vi "Read Input Registers.vi"(8 "error in (no error)":errorcluster, 9 "number of input registers":u16, 10 "address":u16, 11 "MODBUS in":refnum<class "PL Modbus Client.lvclass">) -> (0 "error out":errorcluster, 2 "values":u16[](array[numeric]), 3 "MODBUS out":refnum<class "PL Modbus Client.lvclass">)   [LabVIEW 2015, in "PL Modbus Client.lvclass"]
doc: "Reads a specified <B>number of input registers</B> starting at specified <B>address</B> (Modbus function code: <B>4</B>)."
uses:
  PL Modbus Client.lvclass
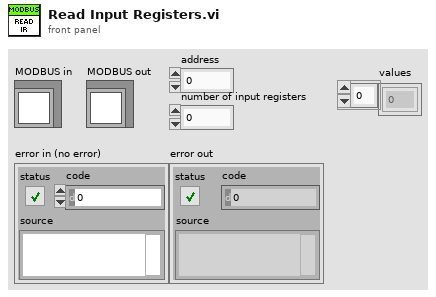
[diagram p1: front panel]
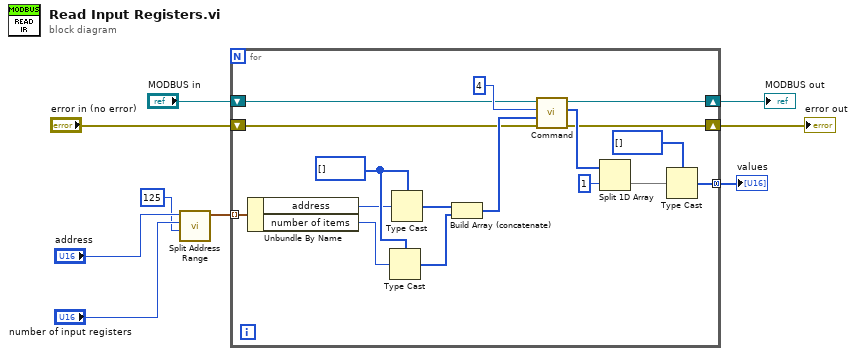
[diagram p0: block diagram]
diagram:
  n1 = call "Split Address Range.vi"("max number of items"=u16 125, "number of items"="number of input registers", "address"="address") -> ("addresses and numbers of items"=w4:cluster{"address":u16, "number of items":u16}[])  [unwired: 8 in]
  n2 = for {
    tunnel: [w12] -> w3 mode=concatenating
    shift-right: [w15] -> w8
    shift-left: "MODBUS in" -> [w16]
    shift-right: [w14] -> w1
    shift-left: "error in (no error)" -> [w13]
    tunnel: w4 -> [w26] mode=indexing
    w17 = u8[] []
    n3 = Unbundle By Name(w26) -> ("address"=w11:u16, "number of items"=w10:u16)
    n4 = Type Cast(type=w17, x=w10) -> (*(type *) &x=w19:u8[])
    n5 = Type Cast(type=w17, x=w11) -> (*(type *) &x=w18:u8[])
    n6 = Build Array (concatenate)(w18, w19) -> (w20:u8[])
    n7 = call-dynamic "Command.vi"("error in (no error)"=w13, "data in"=w20, "function code"=u8 4 ("function"), "MODBUS in"=w16) -> ("error out"=w14:errorcluster, "data out"=w22:u8[], "MODBUS out"=w15:refnum<class "PL Modbus Client.lvclass">)  [unwired: 5 in]
    n8 = Split 1D Array(array=w22, index=1) -> (second subarray=w24:u8[])  [unwired: 1 out]
    n9 = Type Cast(type=u16[] [] ("registers"), x=w24) -> (*(type *) &x=w12:u16[])
  }
  "values" <- w3
  "MODBUS out" <- w8
  "error out" <- w1
